vi "EasyAcquire.IDeviceManager.vi"(11 "Automation Refnum in":refnum<k7>) -> (0 "error out":errorcluster, 1 "hWnd":u32, 2 "GetCurrentDevice":refnum<k7>, 3 "Automation Refnum out":refnum<k7>)   [LabVIEW 2017]
uses:
  C:/Windows/System32/user32.dll
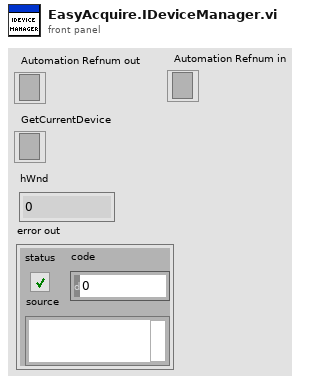
[diagram p1: front panel]
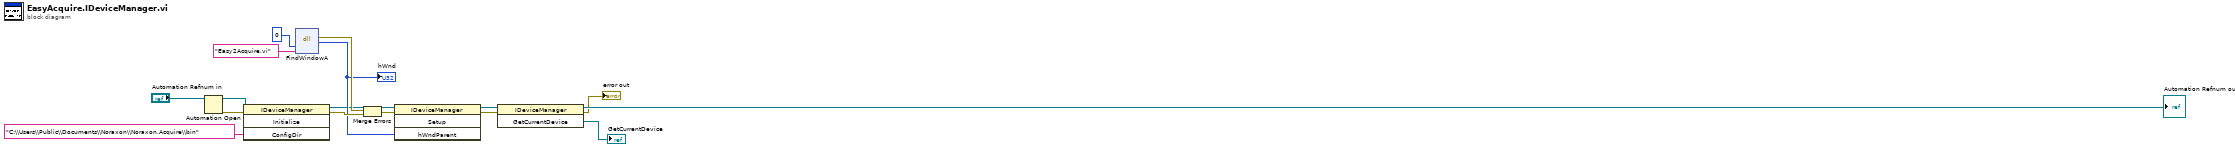
[diagram p0: block diagram]
diagram:
  n1 = Automation Open(Automation Refnum="Automation Refnum in") -> (Automation Refnum=w5:refnum<k7>, error out=w6:errorcluster)  [unwired: 3 in]
  n2 = invoke class="IDeviceManager" method="Initialize"(reference=w5, error in=w6, "ConfigDir"="C:\\Users\\Public\\Documents\\Noraxon\\Noraxon.Acquire\\bin") -> (reference out=w9:refnum<k7>, error out=w13:errorcluster)  [unwired: 1 in, 2 out]
  n3 = dll-call lib="C:/Windows/System32/user32.dll" fn="FindWindowA"("lpszClassName"=0, "lpszWindowName"="Easy2Acquire.vi") -> (error out=w14:errorcluster, "hWnd"=w11:u32)  [unwired: 5 in, 1 out]
  "hWnd" <- w11
  n4 = Merge Errors(w14, w13) -> (w15:errorcluster)
  n5 = invoke class="IDeviceManager" method="Setup"(reference=w9, error in=w15, "hWndParent"=w11) -> (reference out=w10:refnum<k7>, error out=w12:errorcluster)  [unwired: 1 in, 2 out]
  n6 = invoke class="IDeviceManager" method="GetCurrentDevice"(reference=w10, error in=w12) -> (reference out=→"Automation Refnum out":refnum<k7>, error out=→"error out":errorcluster, "GetCurrentDevice"=→"GetCurrentDevice":refnum<k7>)  [unwired: 1 in]
